vi "ConfigureAdvancedSequencer.vi"(3 "error in (no error)":errorcluster, 4 "Advanced Sequencer":T1(array[cluster])=[{"Entry Length"=16384, "Repetition Count"=1, "Infinite Repetitions"=FALSE, "Channels"=[{"Analog Waveform"="SINE", "Amplitude [V]"=2.0, "Offset [V]"=0.0}, {"Analog Waveform"="SINE", "Amplitude [V]"=2.0, "Offset [V]"=0.0}], "Digital Waveform"="", "Wait Event"=1, "Jump Event"=0, "Jump To Mode"=2, "Jump To Entry Item (N)"=1, "Go To Mode"=2, "Go To Entry Item (N)"=1, "Pattern Mode"=2, "Pattern Code"=1, "Pattern Jump To Entry Item (N)"=1, "Pattern Event"=0}] {"Pattern Event" items=["Pattern", "Ext.Mod."]; "Pattern Jump To Entry Item (N)" min=1; "Pattern Code" min=1; "Pattern Mode" items=["First", "Previous", "Next", "Last", "Item"]; "Go To Entry Item (N)" min=1; "Go To Mode" items=["First", "Previous", "Next", "Last", "Item"]; "Jump To Entry Item (N)" min=1; "Jump To Mode" items=["First", "Previous", "Next", "Last", "Item"]; "Jump Event" items=["None", "Button", "Timer", "External", "Ext.Mod."]; "Wait Event" items=["None", "Button", "Timer", "External", "Ext.Mod."]; "Repetition Count" min=1}, 5 "VISA resource name":refnum<visa-resource-name>) -> (0 "error out":errorcluster, 2 "VISA resource name out":refnum<visa-resource-name>)   [LabVIEW 2020, in "Active Technologies AWG3000.lvlib"]
uses:
  Active Technologies AWG3000.lvlib
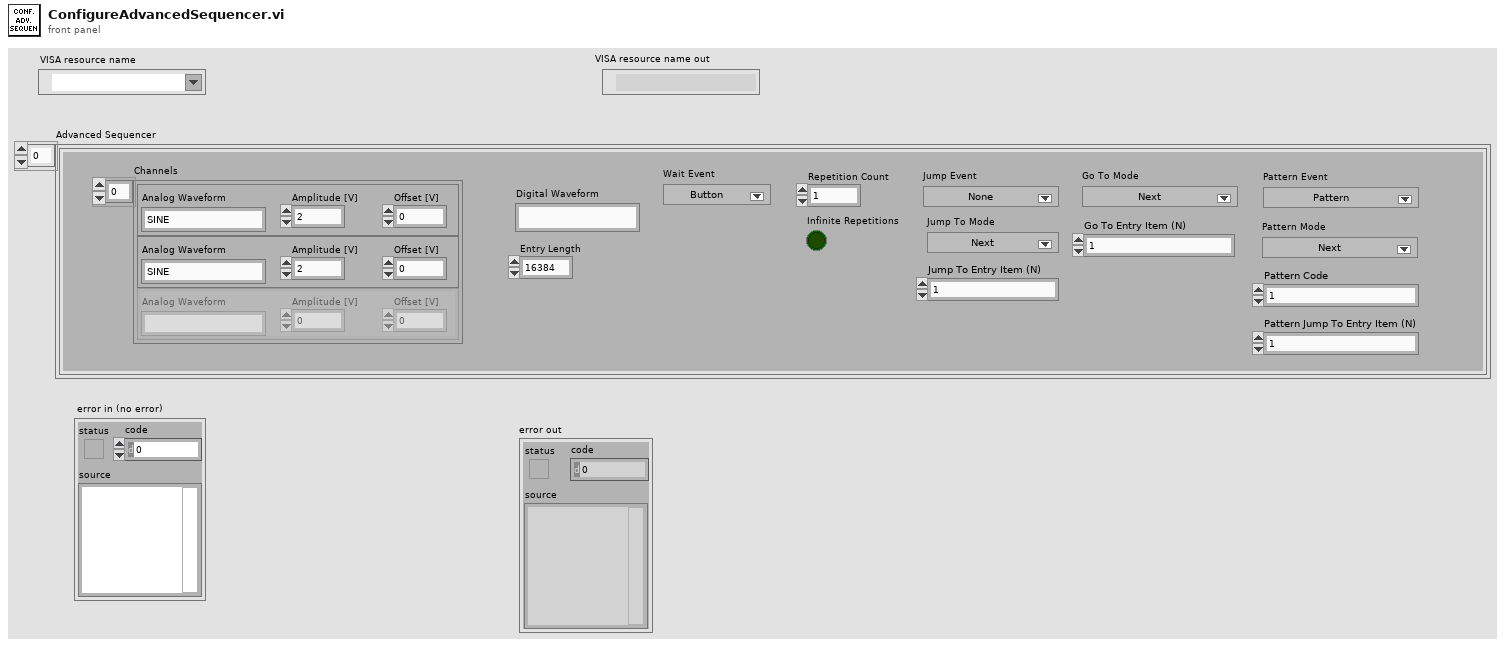
[diagram p1: front panel]
types:
  T1 = cluster{"Entry Length":i32, "Repetition Count":i32, "Infinite Repetitions":bool, "Channels":cluster{"Analog Waveform":string, "Amplitude [V]":dbl, "Offset [V]":dbl}[], "Digital Waveform":string, "Wait Event":u16, "Jump Event":u16, "Jump To Mode":u16, "Jump To Entry Item (N)":i32, "Go To Mode":u16, "Go To Entry Item (N)":i32, "Pattern Mode":u16, "Pattern Code":u8, "Pattern Jump To Entry Item (N)":i32, "Pattern Event":u16}[]
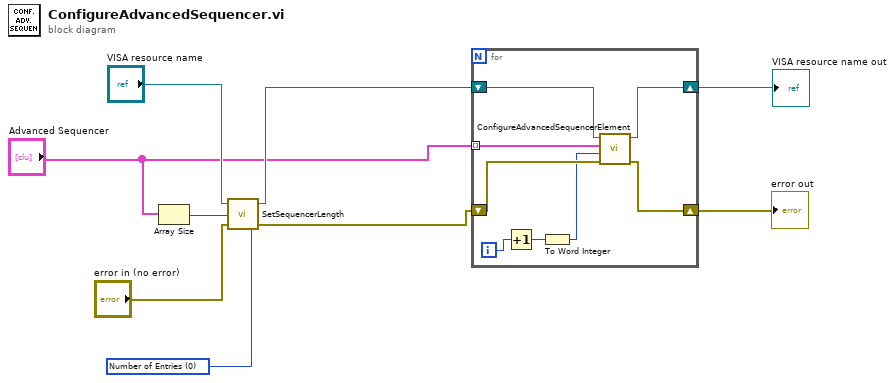
[diagram p0: block diagram]
diagram:
  w4 = u16 0 items=["Number of Entries", "Default", "Minimum", "Maximum"] ("Sequencer Length Options")
  n1 = Array Size(array="Advanced Sequencer") -> (size(s)=w5:i32)
  n2 = call "SetSequencerLength.vi"("Sequencer Length Options"=w4, "error in (no error)"="error in (no error)", "Number of Entries"=w5, "VISA resource name"="VISA resource name") -> ("error out"=w2:errorcluster, "VISA resource name out"=w3:refnum<visa-resource-name>)
  n3 = for {
    shift-right: [w16] -> w9
    shift-left: w3 -> [w17]
    shift-right: [w14] -> w8
    shift-left: w2 -> [w15]
    tunnel: "Advanced Sequencer" -> [w10] mode=indexing
    i -> [w13]
    n4 = Increment(x=w13) -> (x+1=w12:i32)
    n5 = To Word Integer(number=w12) -> (16bit integer=w11:i16)
    n6 = call "ConfigureAdvancedSequencerElement.vi"("error in (no error)"=w15, "Sequencer Element"=w11, "Advanced Sequencer Item"=w10, "VISA resource name"=w17) -> ("error out"=w14:errorcluster, "VISA resource name out"=w16:refnum<visa-resource-name>)  [unwired: 2 in]
  }
  "VISA resource name out" <- w9
  "error out" <- w8
